vi "CSV Parsing.vi"() -> (2 "Files in Directory":path[](array[path]), 3 "CSV Data":string[][][](array[string]))   [LabVIEW 2016]
uses:
  <vilib>/Utility/sysdir.llb/System Directory Type.ctl
  <vilib>/Utility/file.llb/Read Delimited Spreadsheet (string).vi
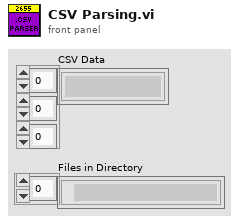
[diagram p1: front panel]
types:
  T1 = typedef "System Directory Type.ctl" = i32
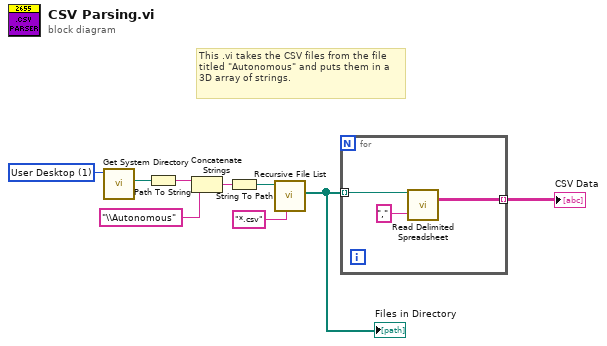
[diagram p0: block diagram]
diagram:
  w7 = T1 1 items=["User Home"=0, "User Desktop"=1, "User Documents"=2, "User Application Data"=3, "User Preferences"=4, "User Temporary"=5, "Public Documents"=6, "Public Application Data"=7, "Public Preferences"=8, "Public Cache"=13, "System Core Libraries"=9, "System Installed Libraries"=10, "Application Files"=11, "Boot Volume Root"=12] ("system directory type")
  # "This .vi takes the CSV files from the file titled \"Autonomous\" and puts them in a 3D array of strings."
  n1 = call <vilib>:"Get System Directory.vi"("system directory type"=w7) -> ("system directory"=w6:path)  [unwired: 10 in]
  n2 = Path To String(path=w6) -> (string=w5:string)
  n3 = Concatenate Strings(w5, "\\Autonomous" ("string")) -> (w3:string)
  n4 = String To Path(string=w3) -> (path=w4:path)
  n5 = call <vilib>:"Recursive File List.vi"("pattern"="*.csv", "Folder Path"=w4) -> ("All Files in Dir"=w8:path[])  [unwired: 5 in, 4 out]
  "Files in Directory" <- w8
  n6 = for {
    tunnel: [w11] -> w9 mode=indexing
    tunnel: w8 -> [w10] mode=indexing
    n7 = call-poly <vilib>:"Read Delimited Spreadsheet.vi"("file path (dialog if empty)"=w10, "delimiter (\\t)"="," ("delimiter (\\t)")) -> ("all rows"=w11:string[][])  [unwired: 8 in, 5 out]
  }
  "CSV Data" <- w9
